vi "Revision number depth.vi"(9 "Depth (2)":u8=2 min=1 max=4, 11 "Full software Revision Number":string="1.2.3.4.5.6") -> (3 "Software Revision Number (first 2 levels only)":string)   [LabVIEW 2020]
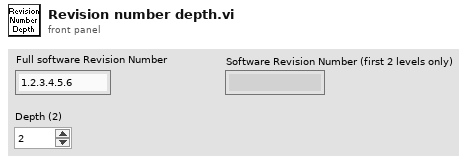
[diagram p1: front panel]
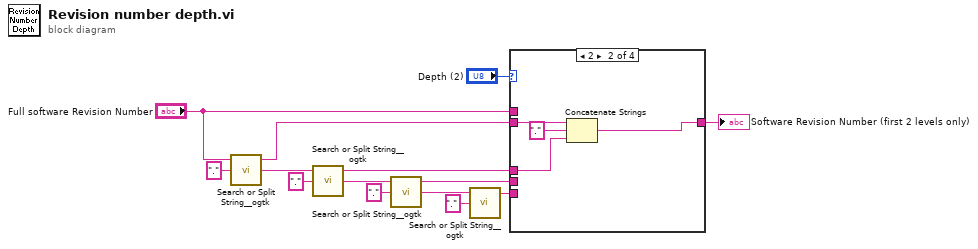
[diagram p0: block diagram]
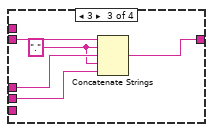
[diagram p3: hidden frame]
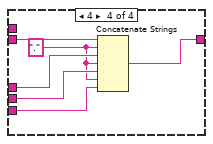
[diagram p4: hidden frame]
diagram:
  n1 = call <userlib>:"Search or Split String__ogtk.vi"("search string/char (-)"=".", "string"="Full software Revision Number") -> ("substring after match"=w13:string, "substring before match"=w11:string)  [unwired: 1 in, 1 out]
  n2 = call <userlib>:"Search or Split String__ogtk.vi"("search string/char (-)"=".", "string"=w13) -> ("substring after match"=w2:string, "substring before match"=w6:string)  [unwired: 1 in, 1 out]
  n3 = call <userlib>:"Search or Split String__ogtk.vi"("search string/char (-)"=".", "string"=w2) -> ("substring after match"=w1:string, "substring before match"=w4:string)  [unwired: 1 in, 1 out]
  n4 = call <userlib>:"Search or Split String__ogtk.vi"("search string/char (-)"=".", "string"=w1) -> ("substring before match"=w3:string)  [unwired: 1 in, 2 out]
  n5 = case shown="2" "Depth (2)" {
    tunnel: w11 -> [w15 w19 w24 w30]
    tunnel: w6 -> [_ w17 w23 w29]
    tunnel: [w15 w16 w22 w28] -> w10
    tunnel: "Full software Revision Number" -> [_ _ _ _]
    tunnel: w4 -> [_ _ w20 w27]
    tunnel: w3 -> [_ _ _ w25]
    frame 1, Default {
    }
    frame 2 {
      n6 = Concatenate Strings(w19, "." ("search string/char (-)"), w17) -> (w16:string)
    }
    frame 3 {
      w21 = "." ("search string/char (-)")
      n7 = Concatenate Strings(w24, w21, w23, w21, w20) -> (w22:string)
    }
    frame 4 {
      w26 = "." ("search string/char (-)")
      n8 = Concatenate Strings(w30, w26, w29, w26, w27, w26, w25) -> (w28:string)
    }
  }
  "Software Revision Number (first 2 levels only)" <- w10
